vi "Array Functions Activity.vi"() -> ()   [LabVIEW 2014]
panel:
  out "已删除的部分":dbl[][](array[numeric])
  out "输出数组":dbl[][](array[numeric])
  out "输出数组":dbl[][](array[numeric])
  out "元素索引":i32
  out "二维数组（Integer）":i32[][](array[numeric])
  out "一维数组(DBL)":dbl[](array[numeric])
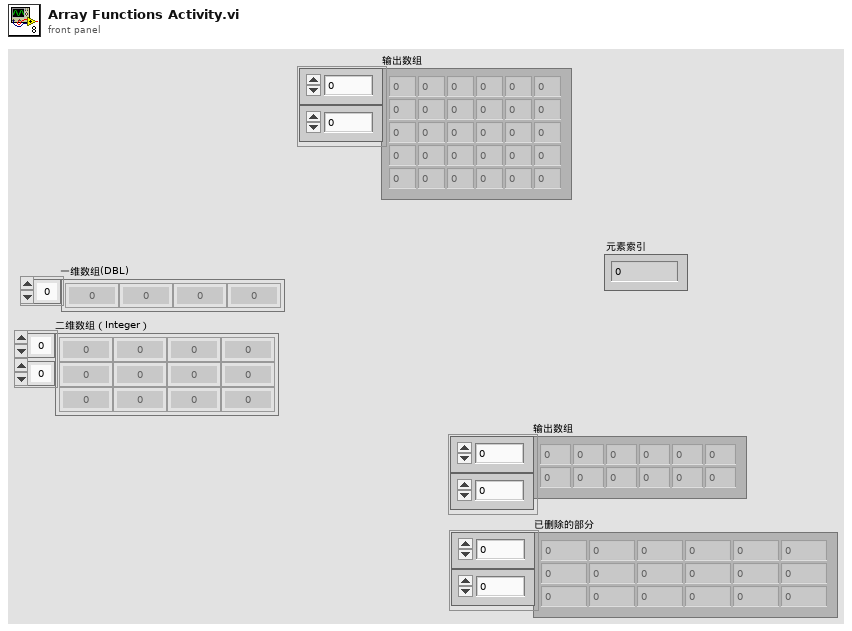
[diagram p1: front panel]
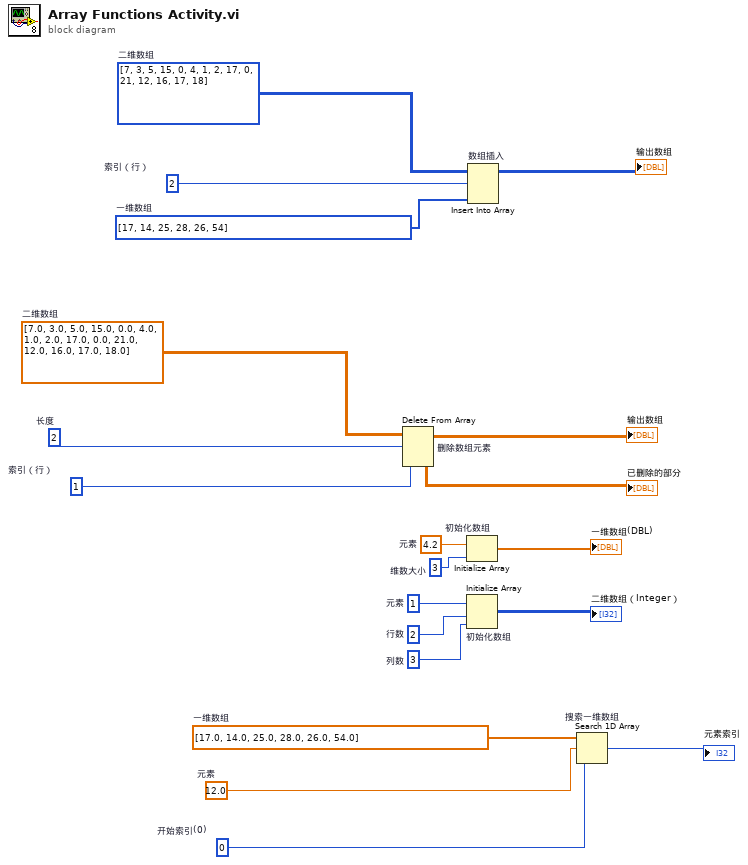
[diagram p0: block diagram]
diagram:
  w3 = 1  # 索引（行）
  w4 = 2  # 长度
  w5 = dbl[][] [[7.0, 3.0, 5.0, 15.0, 0.0], [4.0, 1.0, 2.0, 17.0, 0.0], [21.0, 12.0, 16.0, 17.0, 18.0]]  # 二维数组
  w7 = i32[] [17, 14, 25, 28, 26, 54]  # 一维数组
  w8 = 2  # 索引（行）
  w11 = 0  # 开始索引(0)
  w12 = 12.0  # 元素
  w13 = dbl[] [17.0, 14.0, 25.0, 28.0, 26.0, 54.0]  # 一维数组
  w15 = 3  # 列数
  w16 = 2  # 行数
  w17 = 1  # 元素
  w19 = 3  # 维数大小
  w20 = 4.2  # 元素
  w9 = i32[][] [[7, 3, 5, 15, 0], [4, 1, 2, 17, 0], [21, 12, 16, 17, 18]]  # 二维数组
  n1 = Delete From Array "删除数组元素"(array=w5, length=w4, index (row)=w3) -> (deleted portion=→"已删除的部分":dbl[][], array with subset deleted=→"输出数组":dbl[][])  [unwired: 1 in]
  n2 = Initialize Array "初始化数组"(w20, w19) -> (→"一维数组(DBL)":dbl[])
  n3 = Initialize Array "初始化数组"(w17, w16, w15) -> (→"二维数组（Integer）":i32[][])
  n4 = Insert Into Array "数组插入"(array=w9, index (row)=w8, new element=w7) -> (→"输出数组":i32[][])  [unwired: 1 in]
  n5 = Search 1D Array "搜索一维数组"(1D array=w13, element=w12, start index (0)=w11) -> (index of element=→"元素索引":i32)
